vi "streamFromFile.vi"(8 "error in (no error)":errorcluster, 10 "Path":path, 11 "SoundAO in":refnum<class "SoundAO.lvclass">) -> (0 "error out":errorcluster, 3 "SoundAO out":refnum<class "SoundAO.lvclass">)   [LabVIEW 2011, in "Hardware.lvlib" / "Channels.lvlib" / "SoundAO.lvclass"]
uses:
  SoundAO.lvclass
  AnalogOutput.lvclass
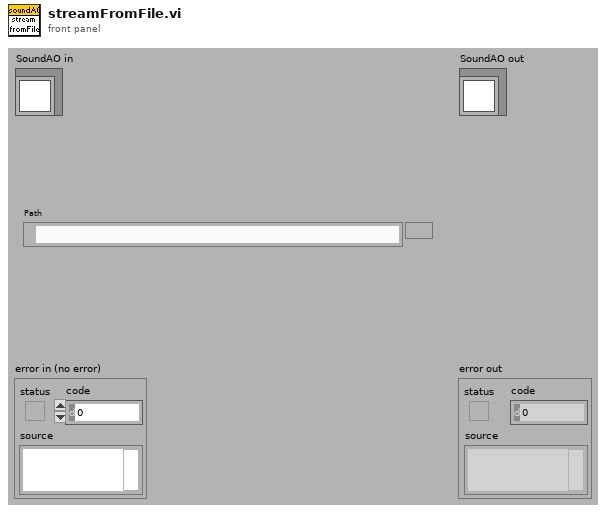
[diagram p1: front panel]
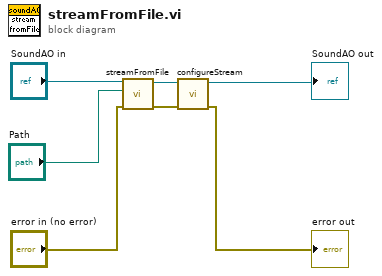
[diagram p0: block diagram]
diagram:
  n1 = call-parent "streamFromFile.vi"("error in (no error)"="error in (no error)", "Path"="Path", "AnalogOutput in"="SoundAO in") -> ("error out"=w3:errorcluster, "AnalogOutput out"=w4:refnum<class "SoundAO.lvclass">)  [unwired: 7 in]
  n2 = call "configureStream.vi"("error in (no error)"=w3, "SoundAO in"=w4) -> ("error out"=→"error out":errorcluster, "SoundAO out"=→"SoundAO out":refnum<class "SoundAO.lvclass">)  [unwired: 8 in]
